vi "Get Buffer Elements.vi"(8 "error in (no error)":errorcluster, 11 "DMM6500 in":refnum<class "DMM6500.lvclass">) -> (0 "error out":errorcluster, 2 "Buffer Elements":string[](array[string])=["CHANNEL", "DATE", "EXTRA", "EXTRAFORMATTED", "EXTRAUNIT", "FORMATTED", "FRACTIONAL", "READING", "RELATIVE", "SECONDS", "STATUS", "TIME", "TSTAMP", "UNIT"], 3 "DMM6500 out":refnum<class "DMM6500.lvclass">)   [LabVIEW 2023, in "HAF.lvlib" / "DMM6500.lvclass"]
doc: "Returns the set of elements that can be used in the DMM6500 buffer."
uses:
  DMM6500.lvclass
  DMM6500.lvclass/DMM6500.ctl
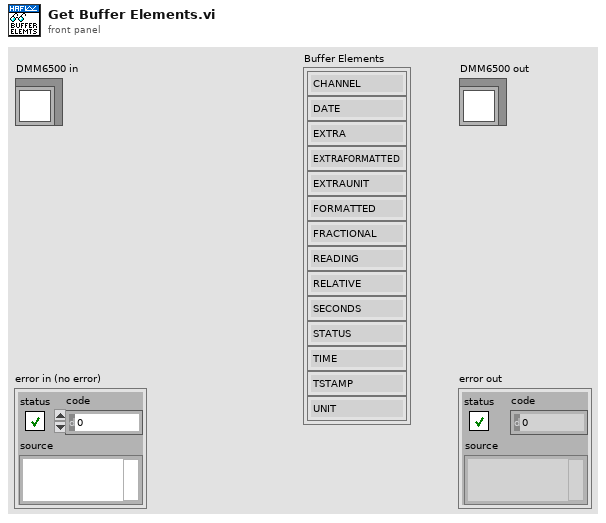
[diagram p1: front panel]
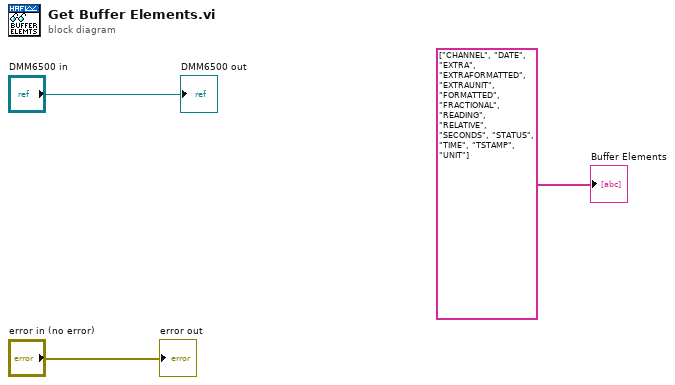
[diagram p0: block diagram]
diagram:
  "error out" <- "error in (no error)"
  "DMM6500 out" <- "DMM6500 in"
  "Buffer Elements" <- string[] ["CHANNEL", "DATE", "EXTRA", "EXTRAFORMATTED", "EXTRAUNIT", "FORMATTED", "FRACTIONAL", "READING", "RELATIVE", "SECONDS", "STATUS", "TIME", "TSTAMP", "UNIT"] ("Buffer Elements")
